vi "Sub_Postprocessing_Timing_Calc.vi"(0 "Experiment In":T1) -> (1 "Experimental Results OUT":T2={"time_average_cycle"=0.0, "measured_frequency"=[], "date_time"="", "estimated_pin_node"=[], "time_cycle_start"=[], "measured_pin_location"=[], "estimated_frequency"=[], "acceleration_data"=[], "accelerometer_sample_rate"=0.0, "displacement_sample_rate"=0.0, "time_compare_start"=array[564 elements], "time_subsample_start"=array[564 elements], "time_FEA_start"=array[564 elements], "time_FEA_end"=array[564 elements], "time_cycle_end"=array[564 elements], "time_accelerometer_aquire_start"=array[564 elements], "time_frequency_calculations_start"=array[564 elements], "time_frequency_calculations_end"=array[564 elements], "measured_pin_location_tt"=array[564 elements], "time_ACC_data_collection_start"=0.0, "time_acceleration_data"=array[564 elements], "estimated_pin_location"=array[564 elements], "scaling_factor_Hz_per_pin_to_frequency_resolution"=1.0, "Std_Dev_equale_particles_divided_3"=TRUE, "Auto_FFT_length"=TRUE, "windowed_acc_data"=array1x564[564 elements], "FFT"=array1x564[564 elements]}, 2 "mean":dbl format="%0.10f")   [LabVIEW 2021]
uses:
  <vilib>/Analysis/baseanly.llb/Mean (DBL).vi
  <vilib>/Analysis/NI_AALBase.lvlib
panel:
  out "number of iterations run":i32
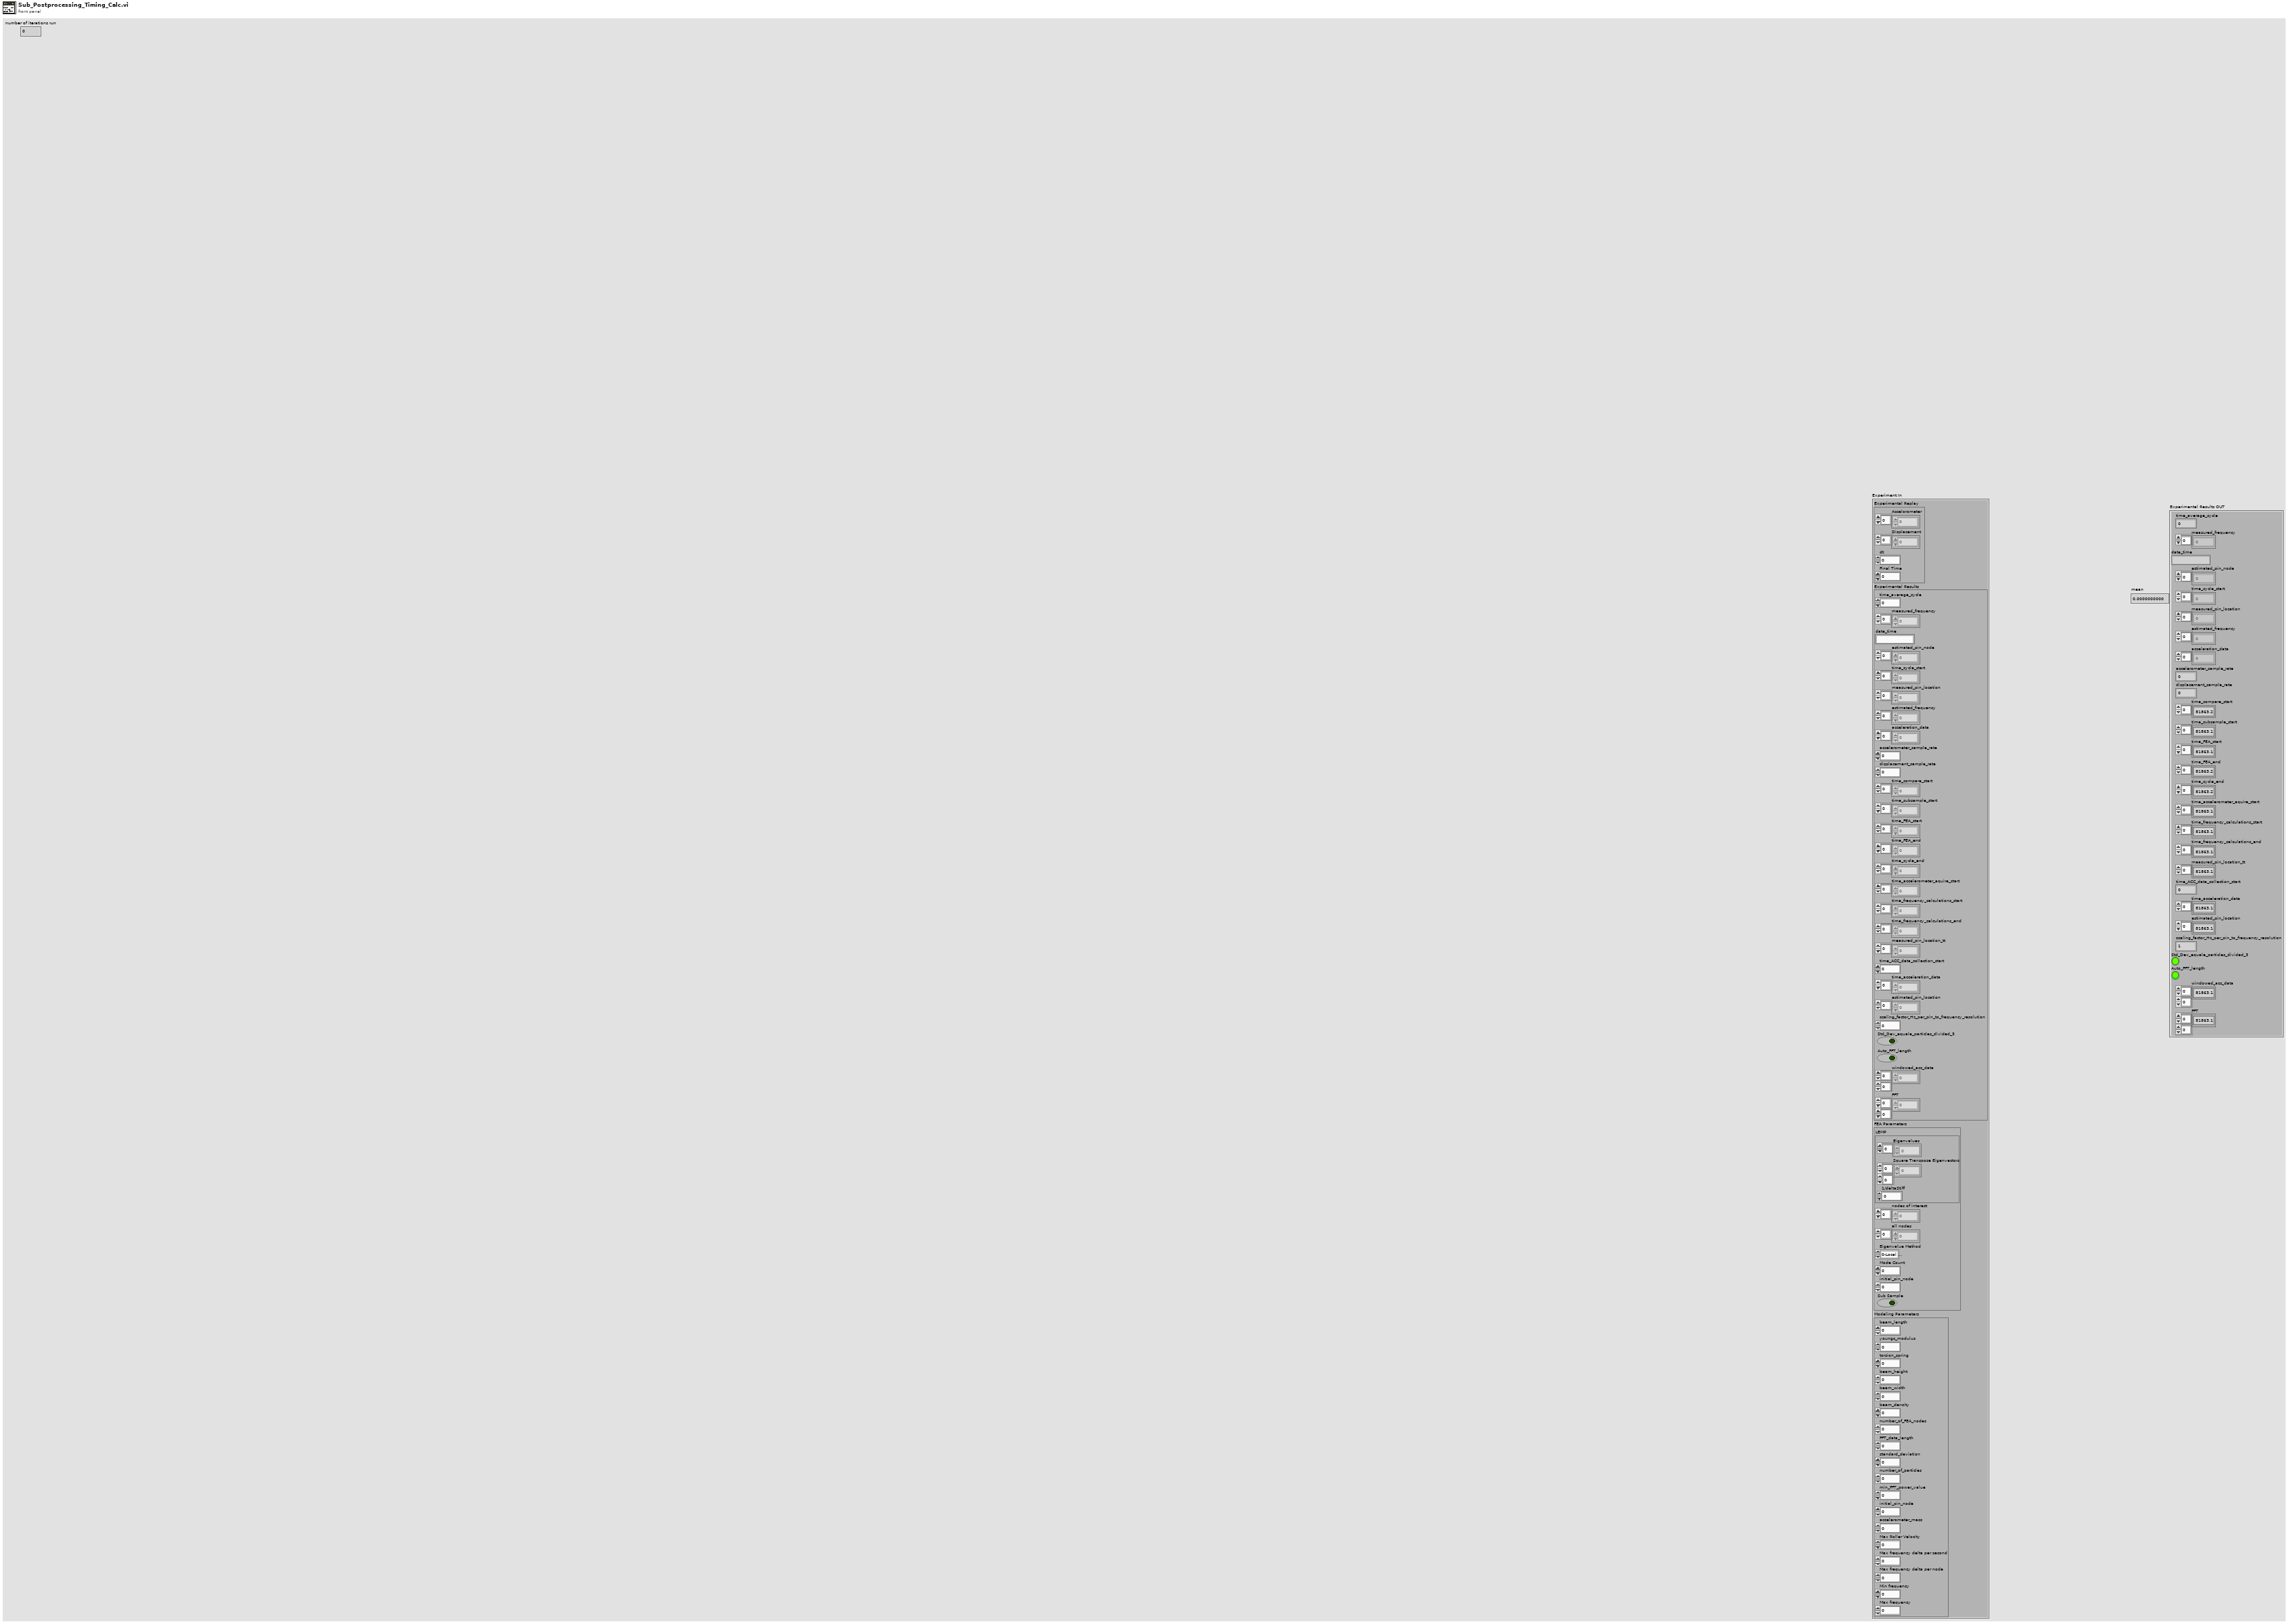
[diagram p1: front panel]
types:
  T1 = cluster{"Experimental Replay":cluster{"Accelorometer":dbl[], "Displacement":dbl[], "dt":dbl, "Final Time":dbl}, "Experimental Results":cluster{"time_average_cycle":dbl, "measured_frequency":dbl[], "date_time":string, "estimated_pin_node":i32[], "time_cycle_start":dbl[], "measured_pin_location":dbl[], "estimated_frequency":dbl[], "acceleration_data":dbl[], "accelerometer_sample_rate":dbl, "displacement_sample_rate":dbl, "time_compare_start":dbl[], "time_subsample_start":dbl[], "time_FEA_start":dbl[], "time_FEA_end":dbl[], "time_cycle_end":dbl[], "time_accelerometer_aquire_start":dbl[], "time_frequency_calculations_start":dbl[], "time_frequency_calculations_end":dbl[], "measured_pin_location_tt":dbl[], "time_ACC_data_collection_start":dbl, "time_acceleration_data":dbl[], "estimated_pin_location":dbl[], "scaling_factor_Hz_per_pin_to_frequency_resolution":dbl, "Std_Dev_equale_particles_divided_3":bool, "Auto_FFT_length":bool, "windowed_acc_data":dbl[][], "FFT":dbl[][]}, "FEA Parameters":cluster{"LEMP":cluster{"Eigenvalues":dbl[], "Square Transpose Eigenvectors":dbl[][], "1/deltaStiff":dbl}, "nodes of interest":i32[], "all nodes":i32[], "Eigenvalue Method":enum16{"0-Local Eigen Modification Procedure", "1-LabVIEW generalized eigenvalues", "2-LabVIEW M^-1K eigenvalues", "3-LabVIEW Cholesky Factorization", "4-Cholesky Factorization CPU SGL", "5-Cholesky Factorization CPU FXP", "6-Cholesky Factorization FPGA SGL", "7-Cholesky Factorization FPGA SGL SCL"}, "Mode Count":i32, "initial_pin_node":i32, "Sub Sample":bool}, "Modeling Parameters":cluster{"beam_length":dbl, "youngs_modulus":dbl, "torsion_spring":dbl, "beam_height":dbl, "beam_width":dbl, "beam_density":dbl, "number_of_FEA_nodes":i32, "FFT_data_length":i32, "standard_deviation":dbl, "number_of_particles":i32, "min_FFT_power_value":dbl, "initial_pin_node":i32, "accelerometer_mass":dbl, "Max Roller Velocity":dbl, "Max frequency delta per second":dbl, "Max frequency delta per node":dbl, "Min frequency":dbl, "Max frequency":dbl}}
  T2 = cluster{"time_average_cycle":dbl, "measured_frequency":dbl[], "date_time":string, "estimated_pin_node":i32[], "time_cycle_start":dbl[], "measured_pin_location":dbl[], "estimated_frequency":dbl[], "acceleration_data":dbl[], "accelerometer_sample_rate":dbl, "displacement_sample_rate":dbl, "time_compare_start":dbl[], "time_subsample_start":dbl[], "time_FEA_start":dbl[], "time_FEA_end":dbl[], "time_cycle_end":dbl[], "time_accelerometer_aquire_start":dbl[], "time_frequency_calculations_start":dbl[], "time_frequency_calculations_end":dbl[], "measured_pin_location_tt":dbl[], "time_ACC_data_collection_start":dbl, "time_acceleration_data":dbl[], "estimated_pin_location":dbl[], "scaling_factor_Hz_per_pin_to_frequency_resolution":dbl, "Std_Dev_equale_particles_divided_3":bool, "Auto_FFT_length":bool, "windowed_acc_data":dbl[][], "FFT":dbl[][]}
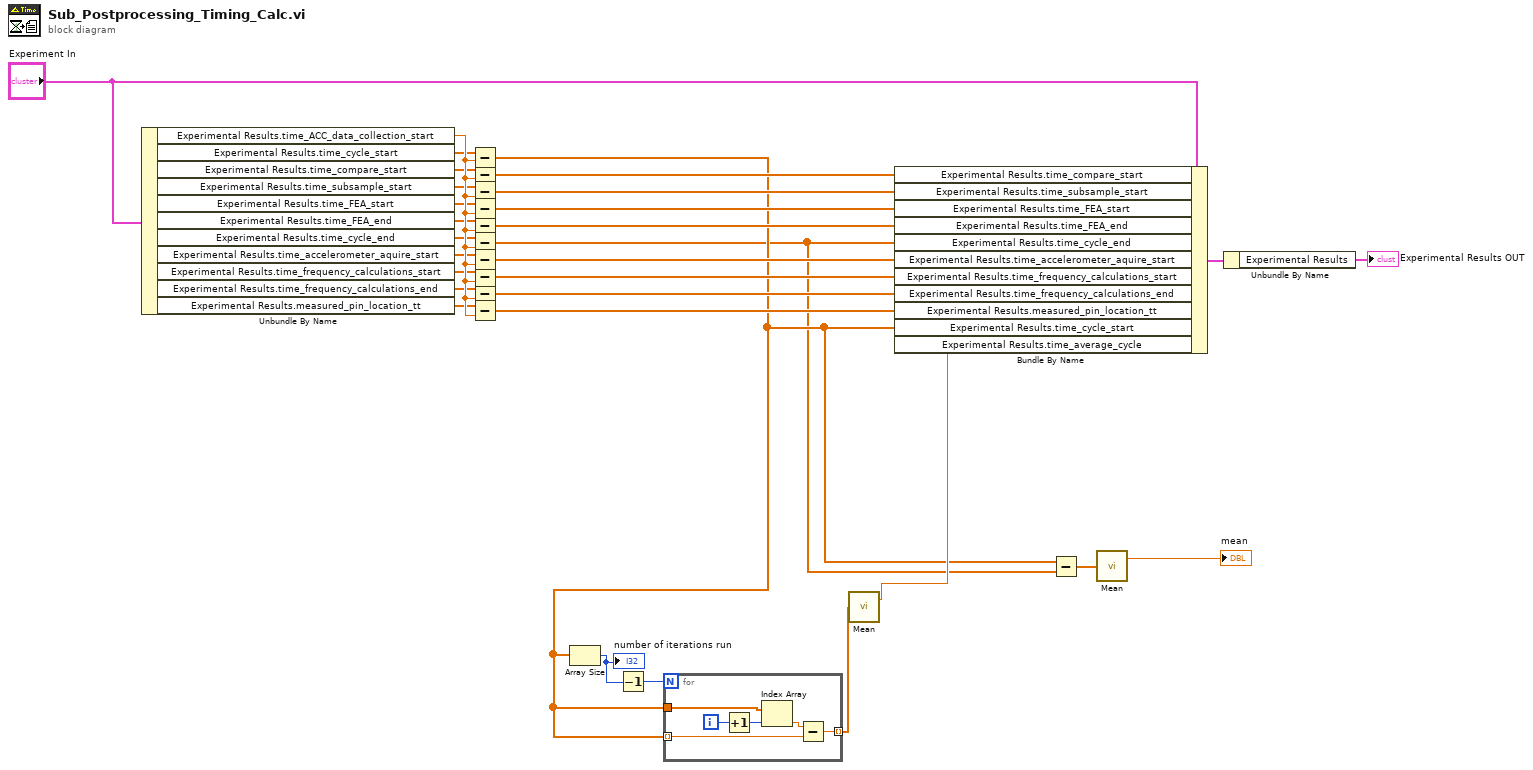
[diagram p0: block diagram]
diagram:
  n1 = Unbundle By Name("Experiment In") -> ("Experimental Results.time_ACC_data_collection_start"=w13:dbl, "Experimental Results.time_cycle_start"=w12:dbl[], "Experimental Results.time_compare_start"=w11:dbl[], "Experimental Results.time_subsample_start"=w10:dbl[], "Experimental Results.time_FEA_start"=w9:dbl[], "Experimental Results.time_FEA_end"=w8:dbl[], "Experimental Results.time_cycle_end"=w7:dbl[], "Experimental Results.time_accelerometer_aquire_start"=w3:dbl[], "Experimental Results.time_frequency_calculations_start"=w4:dbl[], "Experimental Results.time_frequency_calculations_end"=w5:dbl[], "Experimental Results.measured_pin_location_tt"=w6:dbl[])
  n2 = Subtract(x=w12, y=w13) -> (x-y=w2:dbl[])
  n3 = Subtract(x=w11, y=w13) -> (x-y=w30:dbl[])
  n4 = Subtract(x=w10, y=w13) -> (x-y=w29:dbl[])
  n5 = Subtract(x=w9, y=w13) -> (x-y=w28:dbl[])
  n6 = Subtract(x=w8, y=w13) -> (x-y=w25:dbl[])
  n7 = Subtract(x=w7, y=w13) -> (x-y=w1:dbl[])
  n8 = Subtract(x=w3, y=w13) -> (x-y=w27:dbl[])
  n9 = Subtract(x=w4, y=w13) -> (x-y=w19:dbl[])
  n10 = Subtract(x=w5, y=w13) -> (x-y=w20:dbl[])
  n11 = Subtract(x=w6, y=w13) -> (x-y=w26:dbl[])
  n12 = Array Size(array=w2) -> (size(s)=w23:i32)
  "number of iterations run" <- w23
  n13 = Decrement(x=w23) -> (x-1=w24:i32)
  n14 = for {
    N: w24 -> [_]
    tunnel: w2 -> [w36] mode=indexing
    tunnel: w2 -> [w35]
    tunnel: [w31] -> w22 mode=indexing
    i -> [w34]
    n15 = Increment(x=w34) -> (x+1=w33:i32)
    n16 = Index Array(array=w35, index=w33) -> (element=w32:dbl)
    n17 = Subtract(x=w32, y=w36) -> (x-y=w31:dbl)
  }
  n18 = call-poly <vilib>:"Mean.vi"("X"=w22) -> ("mean"=w21:dbl)  [unwired: 1 out]
  n19 = Bundle By Name(cluster="Experiment In", "Experimental Results.time_compare_start"=w30, "Experimental Results.time_subsample_start"=w29, "Experimental Results.time_FEA_start"=w28, "Experimental Results.time_FEA_end"=w25, "Experimental Results.time_cycle_end"=w1, "Experimental Results.time_accelerometer_aquire_start"=w27, "Experimental Results.time_frequency_calculations_start"=w19, "Experimental Results.time_frequency_calculations_end"=w20, "Experimental Results.measured_pin_location_tt"=w26, "Experimental Results.time_cycle_start"=w2, "Experimental Results.time_average_cycle"=w21) -> (w15:T1)
  n20 = Subtract(x=w2, y=w1) -> (x-y=w18:dbl[])
  n21 = call-poly <vilib>:"Mean.vi"("X"=w18) -> ("mean"=→"mean":dbl)  [unwired: 1 out]
  n22 = Unbundle By Name(w15) -> ("Experimental Results"=→"Experimental Results OUT":T2)
